vi "U64.vi"(4 "Value":u64) -> (1 "Constant":refnum<class "Const_U64.lvclass">)   [LabVIEW 2021, in "Const_U64.lvclass"]
uses:
  Const_U64.lvclass
  Const_U64.lvclass/Const_U64.ctl
  Properties/Write Value.vi
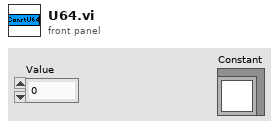
[diagram p1: front panel]
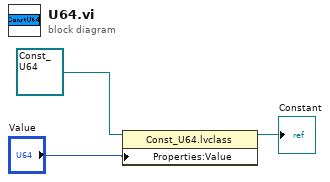
[diagram p0: block diagram]
diagram:
  n1 = property class="Const_U64.lvclass"(reference=refnum<class "Const_U64.lvclass"> refnum ("Constants.lvlib:Numeric.lvclass"), "Properties:Value"="Value") -> (reference out=→"Constant":refnum<class "Const_U64.lvclass">)  [unwired: 1 in, 1 out]
